vi "main.vi"() -> ()   [LabVIEW 2015]
panel:
  out "Result":string="Test123\nHer skal \nkoden til NI scope være."
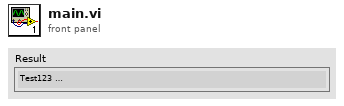
[diagram p1: front panel]
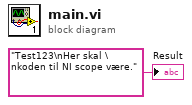
[diagram p0: block diagram]
diagram:
  "Result" <- "Test123\nHer skal \nkoden til NI scope være."
